vi "Create Engine Stream Refs.vi"(6 "Termination":u32(ring) items=["Off", "On"], 7 "Default IDs":u32[](array[numeric]), 8 "error in (no error)":errorcluster, 9 "Cluster":refnum<k21>, 10 "Port":refnum<k21>, 11 "Addon":string) -> (0 "error out":errorcluster, 3 "Refs":T1 {"Termination" items=["Off", "On"]})   [LabVIEW 2019, in "CAN Streaming Support Engine.lvlib"]
uses:
  CAN Streaming Support Engine.lvlib
  Types/Engine Stream API Refs.ctl
  Addon Shared/Types/Direction Filter.ctl
  Addon Shared/Types/Type Filter.ctl
  Addon Shared/Types/Filter Parameters.ctl
  Addon Shared/CAN Streaming Support Shared.lvlib
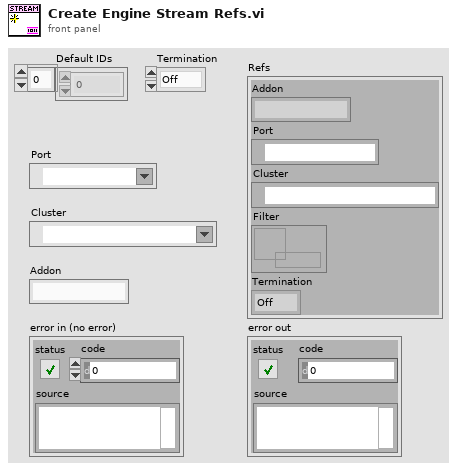
[diagram p1: front panel]
types:
  T1 = typedef "CAN Streaming Support Engine.lvlib/Engine Stream API Refs.ctl" = cluster{"Addon":string, "Port":refnum<k21>, "Cluster":refnum<k21>, "Filter":refnum<data-value>, "Termination":u32}
  T2 = typedef "CAN Streaming Support Shared.lvlib/Filter Parameters.ctl" = cluster{"ID Filters":u32[], "Direction Filter":T3, "Type Filter":T4}
  T3 = typedef "CAN Streaming Support Shared.lvlib/Direction Filter.ctl" = enum16{"Tx/Rx", "Rx", "Tx"}
  T4 = typedef "CAN Streaming Support Shared.lvlib/Type Filter.ctl" = enum16{"All", "CAN Data", "CAN Remote", "CAN Bus Error", "CAN 2.0 Data", "CAN FD Data", "CAN FD+BRS Data", "J1939 Data", "Delay", "Log Trigger", "Start Trigger"}
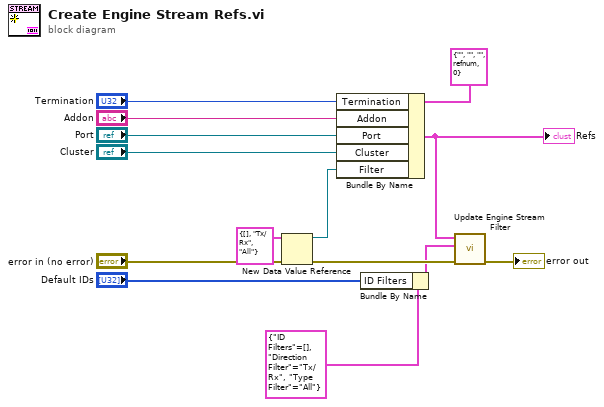
[diagram p0: block diagram]
diagram:
  n1 = New Data Value Reference(data value=T2 {"ID Filters"=[], "Direction Filter"=enum."Tx/Rx", "Type Filter"=enum."All"}, error in="error in (no error)") -> (data value reference=w4:refnum<data-value>, error out=w7:errorcluster)
  n2 = Bundle By Name(cluster=T1 {"Addon"="", "Port"="", "Cluster"="", "Filter"=refnum, "Termination"=0}, "Termination"="Termination", "Addon"="Addon", "Port"="Port", "Cluster"="Cluster", "Filter"=w4) -> (w8:T1)
  "Refs" <- w8
  n3 = Bundle By Name(cluster=T2 {"ID Filters"=[], "Direction Filter"=enum."Tx/Rx", "Type Filter"=enum."All"} ("Filter"), "ID Filters"="Default IDs") -> (w2:T2)
  n4 = call "Update Engine Stream Filter.vi"("error in (no error)"=w7, "Filter"=w2, "Refs"=w8) -> ("error out"=→"error out":errorcluster)  [unwired: 8 in]
